vi "Archive Data.vi"(8 "error in (no error)":errorcluster, 11 "System Configuration":T1) -> (0 "error out":errorcluster, 3 "Succeed?":bool)   [LabVIEW 2024]
doc: "Archives all data in the logging database to the archive database."
uses:
  Controls/Server/System Configuration.ctl
  Controls/Server/Subsystem Configuration.ctl
  <vilib>/lvdsc/NI_DSC.lvlib
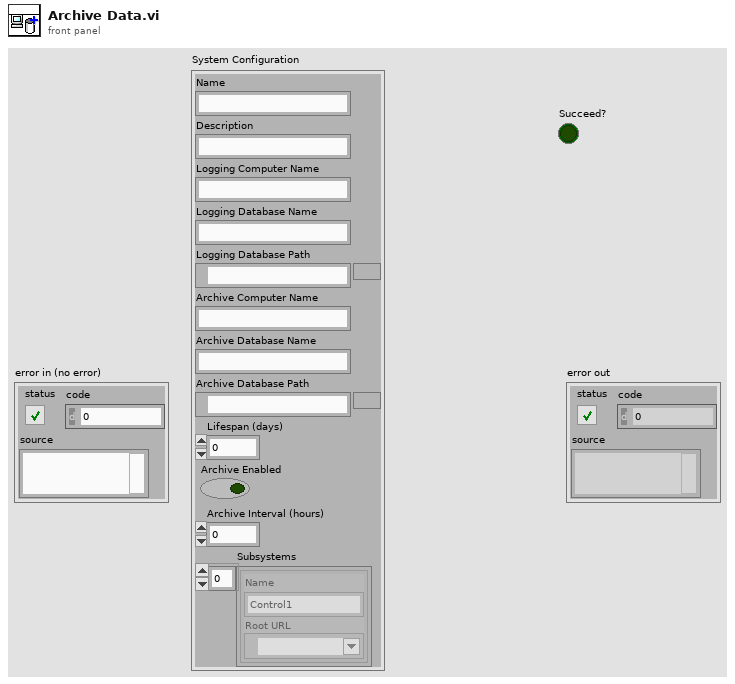
[diagram p1: front panel]
types:
  T1 = typedef "System Configuration.ctl" = cluster{"Name":string, "Description":string, "Logging Computer Name":string, "Logging Database Name":string, "Logging Database Path":path, "Archive Computer Name":string, "Archive Database Name":string, "Archive Database Path":path, "Lifespan (days)":u32, "Archive Enabled":bool, "Archive Interval (hours)":u32, "Subsystems":T2[]}
  T2 = typedef "Subsystem Configuration.ctl" = cluster{"Name":string, "Root URL":refnum<k21>}
  T3 = cluster{"show status bar (T)":bool, "compact (T)":bool, "use * as wildcard (F)":bool, "delete data from source database (F)":bool}
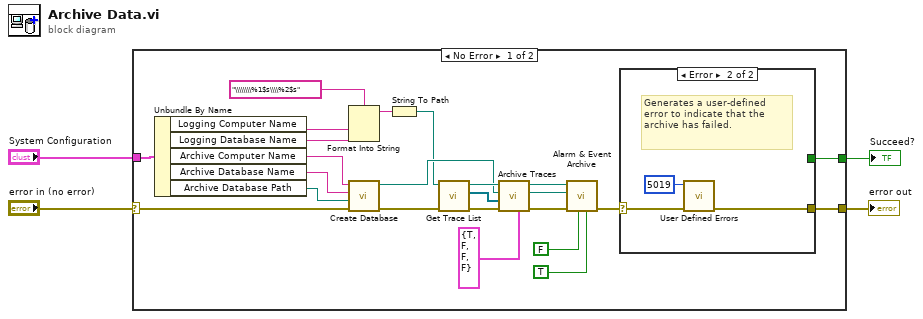
[diagram p0: block diagram]
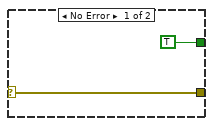
[diagram p2: hidden frame]
diagram:
  n1 = case shown="No Error" "error in (no error)" {
    selector: "error in (no error)" -> [w8 w34]
    tunnel: [w6 w34] -> w4
    tunnel: "System Configuration" -> [w9 _]
    tunnel: [w5 _] -> w1
    frame No Error {
      n2 = Unbundle By Name(w9) -> ("Logging Computer Name"=w15:string, "Logging Database Name"=w14:string, "Archive Computer Name"=w28:string, "Archive Database Name"=w27:string, "Archive Database Path"=w26:path)
      n3 = Format Into String(format string="\\\\\\\\%1$s\\\\%2$s", w15, w14) -> (resulting string=w12:string)  [unwired: 2 in, 1 out]
      n4 = call <vilib>:"Create Database.vi"("error in (no error)"=w8, "database path"=w26, "database name"=w27, "computer name"=w28) -> ("error out"=w10:errorcluster, "database URL out"=w16:path)  [unwired: 4 in, 1 out]
      n5 = String To Path(string=w12) -> (path=w11:path)
      n6 = call <vilib>:"Get Trace List.vi"("error in (no error)"=w10, "database URL"=w11) -> ("error out"=w24:errorcluster, "trace list"=w23:refnum<k21>[], "database URL out"=w25:path)  [unwired: 5 in, 2 out]
      n7 = call <vilib>:"Archive Traces.vi"("options"=T3 {"show status bar (T)"=TRUE, "compact (T)"=FALSE, "use * as wildcard (F)"=FALSE, "delete data from source database (F)"=FALSE}, "error in (no error)"=w24, "trace names"=w23, "destination database URL"=w16, "source database URL"=w25) -> ("error out"=w17:errorcluster, "destination database URL out"=w21:path, "source database URL out"=w22:path)  [unwired: 4 in]
      n8 = call <vilib>:"Alarm & Event Archive.vi"("show status bar (T)"=TRUE, "delete data from\nsource database (F)"=FALSE ("delete data from\nsource database (F)"), "error in (no error)"=w17, "destination database URL"=w21, "source database URL"=w22) -> ("error out"=w7:errorcluster)  [unwired: 4 in, 2 out]
      n9 = case shown="Error" w7 {
        selector: w7 -> [w29 w33]
        tunnel: [w29 w32] -> w6
        tunnel: [TRUE ("Succeed?") _] -> w5
        frame No Error {
        }
        frame Error {
          # "Generates a user-defined error to indicate that the archive has failed."
          n10 = call "User Defined Errors.vi"("error in (no error)"=w33, "Error Code (0)"=5019 ("error code (0)")) -> ("error out"=w32:errorcluster)  [unwired: 9 in]
        }
      }
    }
    frame Error {
    }
  }
  "error out" <- w4
  "Succeed?" <- w1
